vi "DSF.Engine.Execution.Framework.Get Runtime Data.vi"(8 "error in (no error)":errorcluster, 11 "Framework in":refnum<class "DSF.Engine.Execution.Framework.lvclass">) -> (0 "error out":errorcluster, 2 "Framework Runtime Data":T1, 3 "Framework out":refnum<class "DSF.Engine.Execution.Framework.lvclass">)   [LabVIEW 2016, in "DSF.Engine.lvlib" / "DSF.Engine.Execution.Framework.lvclass"]
uses:
  DSF.Engine.Execution.Framework.lvclass
  DSF.Engine.Execution.Framework.Framework Runtime Data.ctl
  DSF.Engine.Execution.Framework.lvclass/DSF.Engine.Execution.Framework.ctl
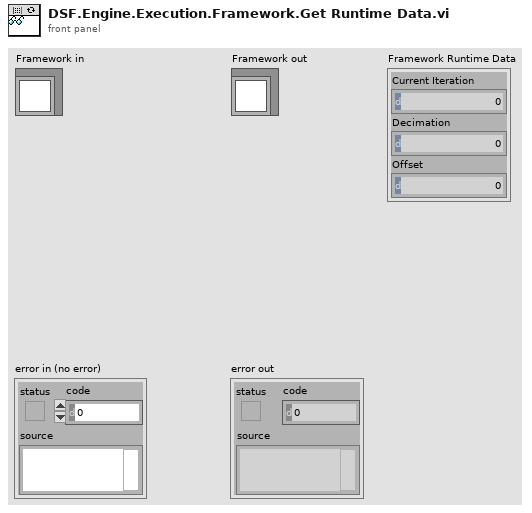
[diagram p1: front panel]
types:
  T1 = typedef "DSF.Engine.lvlib/DSF.Engine.Execution.Framework.lvclass/DSF.Engine.Execution.Framework.Framework Runtime Data.ctl" = cluster{"Current Iteration":u64, "Decimation":u64, "Offset":u64}
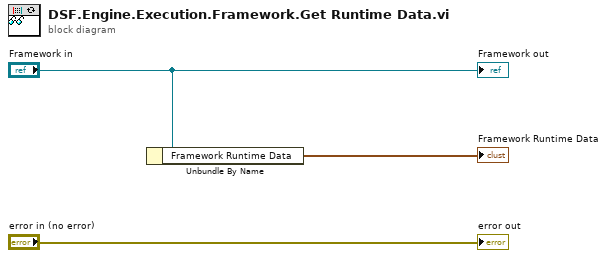
[diagram p0: block diagram]
diagram:
  n1 = Unbundle By Name("Framework in") -> ("Framework Runtime Data"=→"Framework Runtime Data":T1)
  "error out" <- "error in (no error)"
  "Framework out" <- "Framework in"
